vi "Close Report File.vi"(8 "error in (no error)":errorcluster, 11 "Coverage Report In":refnum<class "Coverage Report.lvclass">) -> (0 "error out":errorcluster, 2 "Report Path":path)   [LabVIEW 2020, in "Coverage Report.lvclass"]
uses:
  Coverage Report.lvclass
  Coverage Report.lvclass/Coverage Report.ctl
  8819afad-9df6-4925-b28a-05efd8fb8022.vi
  <vilib>/Platform/browser.llb/Open URL in Default Browser (path).vi
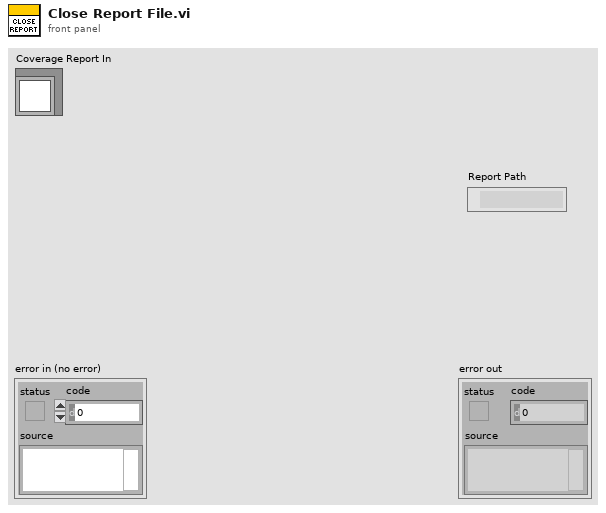
[diagram p1: front panel]
types:
  T1 = enum16{"open", "replace", "create", "open or create", "replace or create", "replace or create with confirmation"}
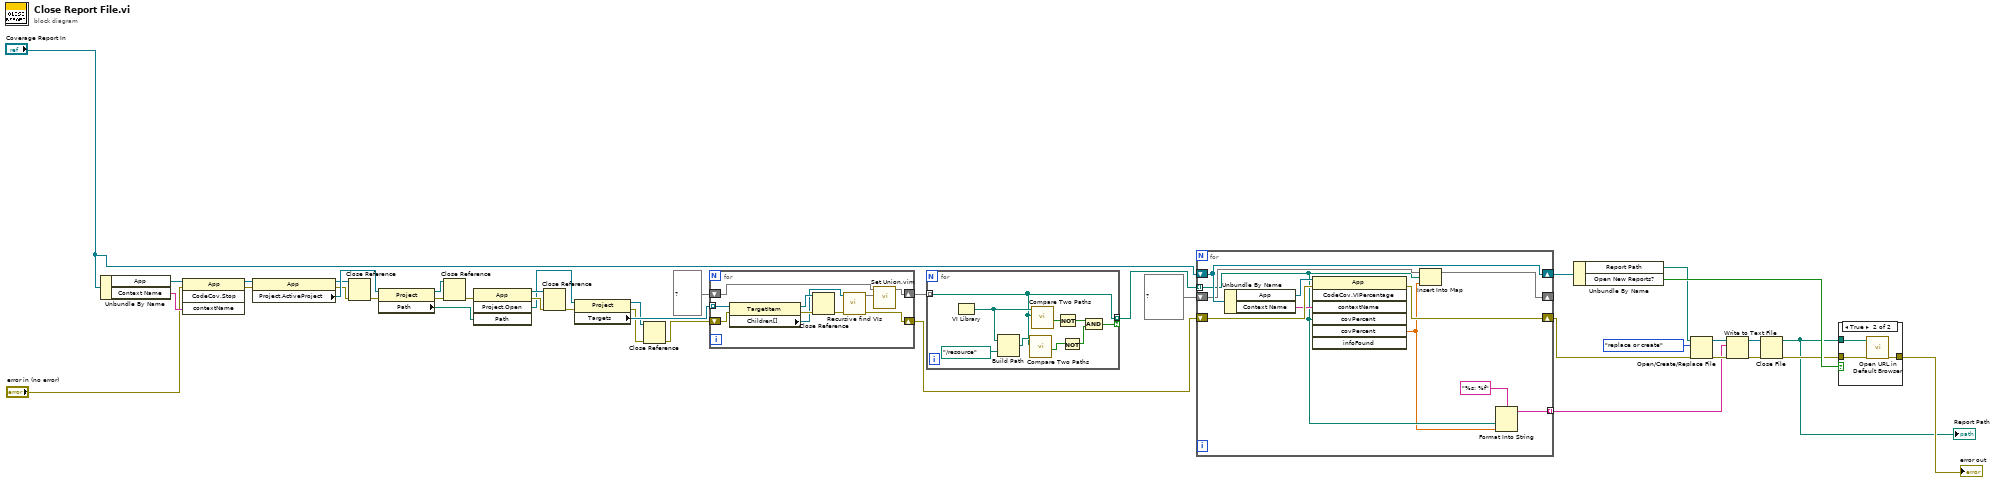
[diagram p0: block diagram]
diagram:
  n1 = Unbundle By Name("Coverage Report In") -> ("App"=w40:refnum<vi>, "Context Name"=w39:string)
  n2 = invoke class="App" method="CodeCov.Stop"(reference=w40, error in="error in (no error)", "contextName"=w39) -> (reference out=w32:refnum<vi>, error out=w29:errorcluster)  [unwired: 1 in, 2 out]
  n3 = property class="App"(reference=w32, error in=w29) -> (reference out=w37:refnum<vi>, error out=w34:errorcluster, "Project.ActiveProject"=w38:refnum<vi>)
  n4 = Close Reference(reference=w37, error in (no error)=w34) -> (error out=w33:errorcluster)
  n5 = property class="Project"(reference=w38, error in=w33) -> (reference out=w36:refnum<vi>, error out=w35:errorcluster, "Path"=w30:path)
  n6 = Close Reference(reference=w36, error in (no error)=w35) -> (error out=w28:errorcluster)
  n7 = invoke class="App" method="Project.Open"(error in=w28, "Path"=w30) -> (reference out=w23:refnum<vi>, error out=w19:errorcluster, "Project:Open"=w17:refnum<vi>)  [unwired: 2 in, 1 out]
  n8 = Close Reference(reference=w23, error in (no error)=w19) -> (error out=w22:errorcluster)
  n9 = property class="Project"(reference=w17, error in=w22) -> (reference out=w21:refnum<vi>, error out=w18:errorcluster, "Targets"=w26:refnum<vi>[])
  n10 = Close Reference(reference=w21, error in (no error)=w18) -> (error out=w20:errorcluster)
  n11 = for {
    tunnel: w26 -> [w50] mode=indexing
    shift-right: [w47] -> w31
    shift-left: w20 -> [w48]
    shift-right: [w43] -> w25
    shift-left: set{path} {} ("VIs") -> [w45]
    n12 = property class="TargetItem"(reference=w50, error in=w48) -> (reference out=w46:refnum<vi>, error out=w49:errorcluster, "Children[]"=w41:refnum<vi>[])
    n13 = Close Reference(reference=w46, error in (no error)=w49) -> (error out=w42:errorcluster)
    n14 = call "Recursive find VIs.vi"("error in (no error)"=w42, "Project Items"=w41) -> ("error out"=w47:errorcluster, "VIs"=w44:set{path})  [unwired: 8 in]
    n15 = call "Set Union.vim"("set 2"=w44, "set 1"=w45) -> ("union"=w43:set{path})  [unwired: 9 in]
  }
  n16 = for {
    tunnel: w25 -> [w51] mode=indexing
    tunnel: [w51] -> w16 mode=indexing if=w56
    n17 = VI Library() -> (path=w54:path)
    n18 = Build Path(base path=w54, name or relative path=path "../resource") -> (appended path=w52:path)
    n19 = call <vilib>:"Compare Two Paths.vi"("Path 2"=w51, "Path 1"=w52) -> ("Path 2 Relative to Path 1?"=w57:bool)  [unwired: 6 in, 3 out]
    n20 = call <vilib>:"Compare Two Paths.vi"("Path 2"=w51, "Path 1"=w54) -> ("Path 2 Relative to Path 1?"=w59:bool)  [unwired: 6 in, 3 out]
    n21 = Not(x=w59) -> (.not. x?=w58:bool)
    n22 = Not(x=w57) -> (.not. x?=w55:bool)
    n23 = And(x=w58, y=w55) -> (x .and. y?=w56:bool)
  }
  n24 = for {
    shift-right: [w70] -> w13
    shift-left: "Coverage Report In" -> [w70]
    shift-right: [w68] -> w5
    shift-left: w31 -> [w69]
    tunnel: w16 -> [w62] mode=indexing
    shift-right: [w66] -> _
    shift-left: map{path, dbl} {} ("Code Coverage") -> [w67]
    tunnel: [w60] -> w1 mode=indexing
    n25 = Unbundle By Name(w70) -> ("App"=w64:refnum<vi>, "Context Name"=w65:string)
    n26 = invoke class="App" method="CodeCov.VIPercentage"(reference=w64, error in=w69, "contextName"=w65, "covPercent"=w62) -> (error out=w68:errorcluster, "covPercent"=w61:dbl)  [unwired: 3 in, 5 out]
    n27 = Insert Into Map(map in=w67, key=w62, value=w61) -> (map out=w66:map{path, dbl})  [unwired: 2 out]
    n28 = Format Into String(format string="%s: %f", w62, w61) -> (resulting string=w60:string)  [unwired: 2 in, 1 out]
  }
  n29 = Unbundle By Name(w13) -> ("Report Path"=w7:path, "Open New Reports?"=w12:bool)
  n30 = Open/Create/Replace File(file path (use dialog)=w7, error in=w5, operation (0:open)=T1."replace or create") -> (refnum out=w11:refnum<file>, error out=w10:errorcluster)  [unwired: 3 in, 1 out]
  n31 = Write to Text File(file (use dialog)=w11, text=w1, error in=w10) -> (refnum out=w9:refnum<file>, error out=w8:errorcluster)  [unwired: 1 in, 1 out]
  n32 = Close File(refnum=w9, error in=w8) -> (path=w3:path, error out=w6:errorcluster)
  "Report Path" <- w3
  n33 = case shown="True" w12 {
    tunnel: w3 -> [_ w72]
    tunnel: w6 -> [w71 w74]
    tunnel: [w71 w73] -> w4
    frame False {
    }
    frame True {
      n34 = call-poly <vilib>:"Open URL in Default Browser.vi"("error in (no error)"=w74, "path"=w72) -> ("error out"=w73:errorcluster)  [unwired: 4 in, 1 out]
    }
  }
  "error out" <- w4
